vi "worksheet repeat columns.vi"(8 "error in (no error)":errorcluster, 9 "last_col":u16, 10 "first_col":u16, 11 "worksheet":u32) -> (0 "error out":errorcluster, 3 "function return":u32(ring))   [LabVIEW 8.6]
doc: "lxw_error worksheet_repeat_columns(lxw_worksheet worksheet, lxw_col_t first_col, lxw_col_t last_col);"
uses:
  pending_lvxlsxwriter/xlsxwriter.dll
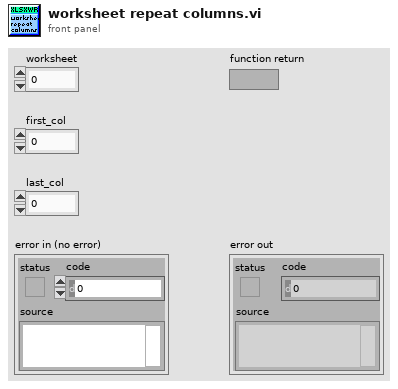
[diagram p1: front panel]
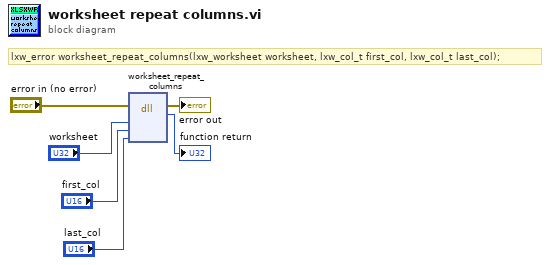
[diagram p0: block diagram]
diagram:
  # "lxw_error worksheet_repeat_columns(lxw_worksheet worksheet, lxw_col_t first_col, lxw_col_t last_col);"
  n1 = dll-call lib="C:/Users/WDAGUtilityAccount/Desktop/pending_lvxlsxwriter/xlsxwriter.*" fn="worksheet_repeat_columns"(error in="error in (no error)", "worksheet"="worksheet", "first_col"="first_col", "last_col"="last_col") -> (error out=→"error out":errorcluster, →"function return":u32)  [unwired: 5 in, 1 out]
